vi "Close.vi"(8 "error in (no error)":errorcluster, 11 "SerialResource in":refnum<class "SerialResource.lvclass">) -> (0 "error out":errorcluster, 3 "SerialResource out":refnum<class "SerialResource.lvclass">)   [LabVIEW 2020]
uses:
  SerialResource.lvclass/SerialResource.ctl
  SerialResource.lvclass
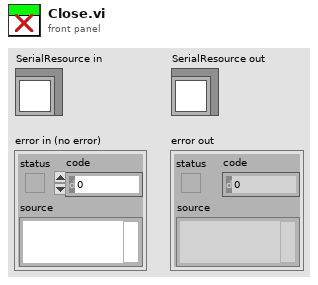
[diagram p1: front panel]
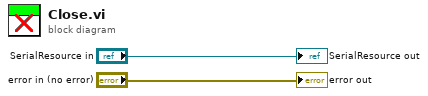
[diagram p0: block diagram]
diagram:
  "error out" <- "error in (no error)"
  "SerialResource out" <- "SerialResource in"
